vi "ExpectedDepsCheckResults.vi"(0 "ResultsArray":T1[](array[typedef]), 5 "Library Name":string, 7 "ExpectedDependencies":string[](array[string]), 9 "ActualDependencies":string[](array[string])) -> (4 "ResultsArray out":T1[](array[typedef]))   [LabVIEW 2023, in "DepsWatch.lvlib"]
uses:
  DepsWatch.lvlib
  Typedefs/DepsCheckResult.ctl
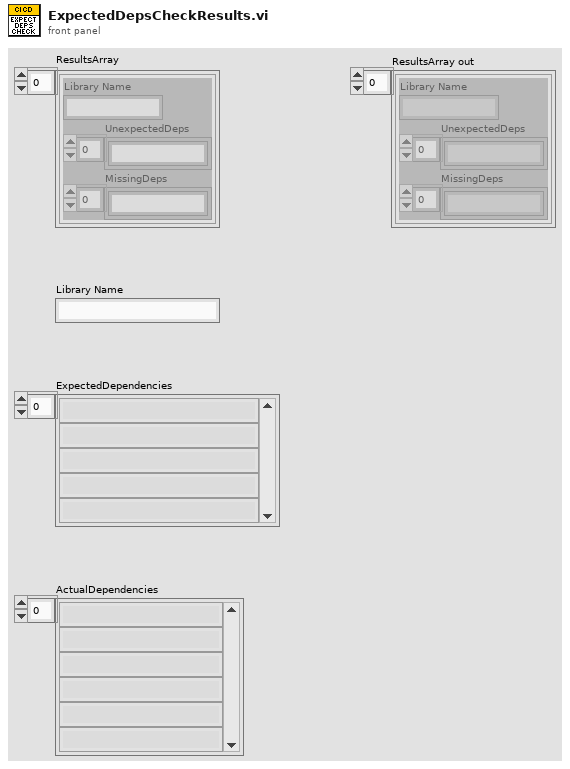
[diagram p1: front panel]
types:
  T1 = typedef "DepsWatch.lvlib/DepsCheckResult.ctl" = cluster{"Library Name":string, "UnexpectedDeps":string[], "MissingDeps":string[]}
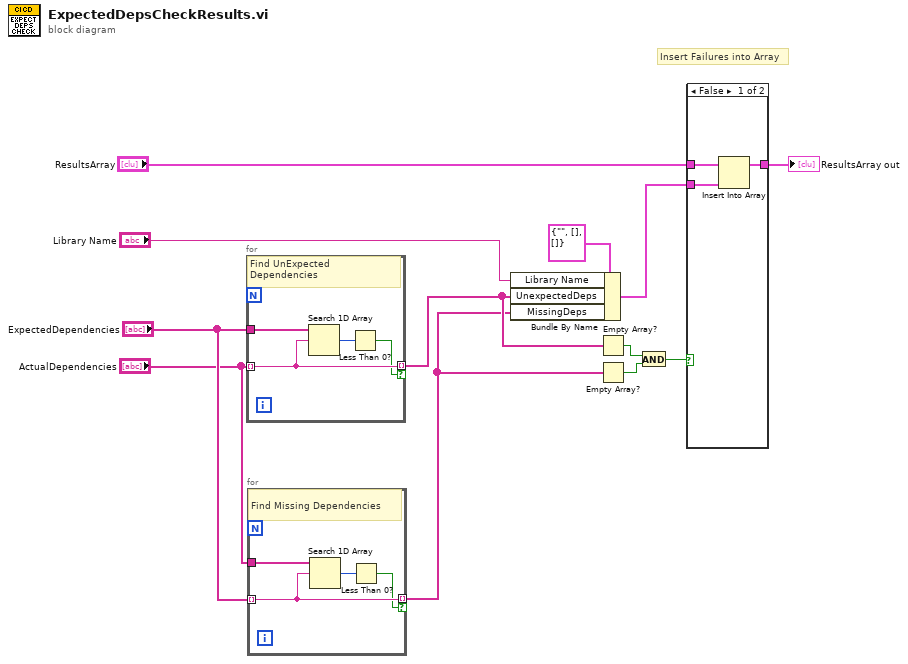
[diagram p0: block diagram]
diagram:
  # "Insert Failures into Array"
  n1 = for {
    tunnel: "ExpectedDependencies" -> [w16]
    tunnel: "ActualDependencies" -> [w14] mode=indexing
    tunnel: [w14] -> w5 mode=indexing if=w13
    # "Find UnExpected Dependencies"
    n2 = Search 1D Array(1D array=w16, element=w14) -> (index of element=w15:i32)  [unwired: 1 in]
    n3 = Less Than 0?(x=w15) -> (x < 0?=w13:bool)
  }
  n4 = for {
    tunnel: "ActualDependencies" -> [w20]
    tunnel: "ExpectedDependencies" -> [w18] mode=indexing
    tunnel: [w18] -> w4 mode=indexing if=w17
    # "Find Missing Dependencies"
    n5 = Search 1D Array(1D array=w20, element=w18) -> (index of element=w19:i32)  [unwired: 1 in]
    n6 = Less Than 0?(x=w19) -> (x < 0?=w17:bool)
  }
  n7 = Bundle By Name(cluster=T1 {"Library Name"="", "UnexpectedDeps"=[], "MissingDeps"=[]}, "Library Name"="Library Name", "UnexpectedDeps"=w5, "MissingDeps"=w4) -> (w7:T1)
  n8 = Empty Array?(array=w5) -> (empty?=w3:bool)
  n9 = Empty Array?(array=w4) -> (empty?=w2:bool)
  n10 = And(x=w3, y=w2) -> (x .and. y?=w1:bool)
  n11 = case shown="False" w1 {
    tunnel: "ResultsArray" -> [w23 w24]
    tunnel: w7 -> [w22 _]
    tunnel: [w21 w24] -> w6
    frame False {
      n12 = Insert Into Array(array=w23, new element=w22) -> (w21:T1[])  [unwired: 1 in]
    }
    frame True {
    }
  }
  "ResultsArray out" <- w6
